vi "Enable Output.vi"(7 "Enable Output (F: Disable)":bool, 8 "error in (no error)":errorcluster, 9 "Operation (0: Set)":i32(ring) items=["Set", "Get"], 10 "Channel (0: Channel 1)":i32(ring) items=["Channel 1", "Channel 2"], 11 "VISA resource name":refnum<visa-resource-name>) -> (0 "error out":errorcluster, 1 "Output Enabled?":bool, 3 "VISA resource name out":refnum<visa-resource-name>)   [LabVIEW 2023, in "Agilent B2900 Series.lvlib"]
doc: "Enables or disables specified output channel.\nCan also query the status of output."
uses:
  Agilent B2900 Series.lvlib
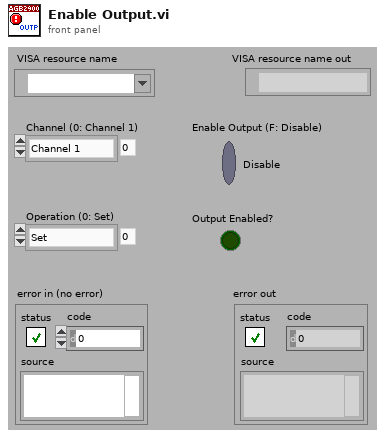
[diagram p1: front panel]
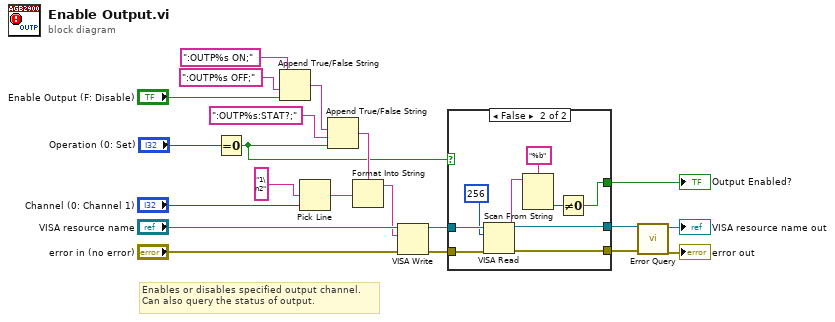
[diagram p0: block diagram]
diagram:
  # "Enables or disables specified output channel.\nCan also query the status of output."
  n1 = Equal To 0?(x="Operation (0: Set)") -> (x = 0?=w2:bool)
  n2 = Append True/False String(1:"Enable Output (F: Disable)", 2:":OUTP%s OFF;", 3:":OUTP%s ON;") -> (0:w4:string)  [unwired: 1 in]
  n3 = Pick Line(multi-line string="1\n2" ("string (\"\")"), line index="Channel (0: Channel 1)") -> (output string=w7:string)  [unwired: 1 in]
  n4 = Append True/False String(1:w2, 2:":OUTP%s:STAT?;" ("format string"), 3:w4) -> (0:w6:string)  [unwired: 1 in]
  n5 = Format Into String(format string=w6, w7) -> (resulting string=w14:string)  [unwired: 2 in, 1 out]
  n6 = VISA Write(VISA resource name="VISA resource name", write buffer=w14, error in (no error)="error in (no error)") -> (VISA resource name out=w11:refnum<visa-resource-name>, error out=w8:errorcluster)  [unwired: 1 out]
  n7 = case shown="False" w2 {
    tunnel: w11 -> [w23 w32]
    tunnel: [w23 w31] -> w10
    tunnel: [w22 w30] -> w9
    tunnel: w8 -> [w22 w29]
    tunnel: [_ w24] -> w1
    frame True {
    }
    frame False {
      n8 = VISA Read(VISA resource name=w32, byte count=u32 256, error in (no error)=w29) -> (VISA resource name out=w31:refnum<visa-resource-name>, read buffer=w27:string, error out=w30:errorcluster)  [unwired: 1 out]
      n9 = Scan From String(format string="%b", input string=w27) -> (output 1=w25:i32)  [unwired: 3 in, 3 out]
      n10 = Not Equal To 0?(x=w25) -> (x != 0?=w24:bool)
    }
  }
  "Output Enabled?" <- w1
  n11 = call "Error Query.vi"("error in (no error)"=w9, "VISA resource name"=w10) -> ("error out"=→"error out":errorcluster, "VISA resource name out"=→"VISA resource name out":refnum<visa-resource-name>)  [unwired: 6 in, 2 out]
